vi "test.vi"() -> ()   [LabVIEW 2017]
uses:
  <vilib>/Instr/_visa.llb/VISA Configure Serial Port (Instr).vi
panel:
  out "返回数 2":u32
  out "返回数":u32
  in  "输入串口（com12）":refnum<visa-resource-name>="COM12"
  out "读取缓冲区1":string="i"
  in  "停止":bool
  in  "输出串口（com13）":refnum<visa-resource-name>="COM13"
  in  "输入串口（com11）":refnum<visa-resource-name>="COM11"
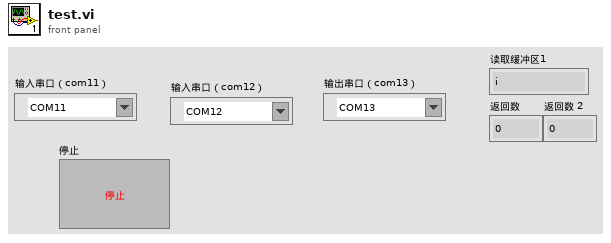
[diagram p1: front panel]
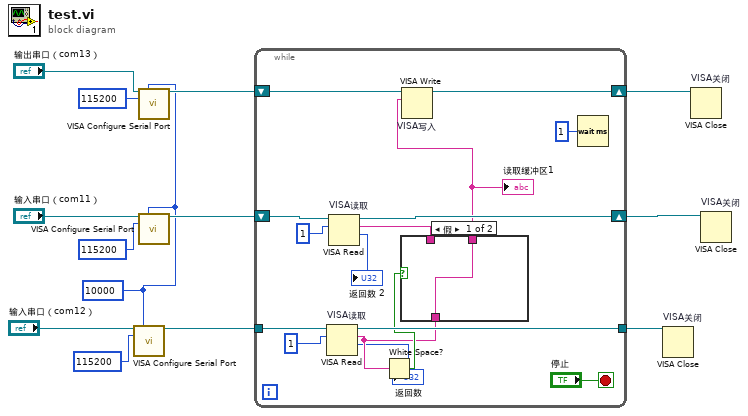
[diagram p0: block diagram]
diagram:
  w1 = u32 10000 ("timeout (10sec)")
  n1 = call-poly "VISA Configure Serial Port"("VISA resource name"="输入串口（com12）", "timeout (10sec)"=w1, "baud rate (9600)"=u32 115200) -> ("VISA resource name out"=w3:refnum<visa-resource-name>)  [unwired: 11 in, 1 out]
  n2 = call-poly "VISA Configure Serial Port"("VISA resource name"="输出串口（com13）", "timeout (10sec)"=w1, "baud rate (9600)"=u32 115200) -> ("VISA resource name out"=w8:refnum<visa-resource-name>)  [unwired: 11 in, 1 out]
  n3 = call-poly "VISA Configure Serial Port"("VISA resource name"="输入串口（com11）", "timeout (10sec)"=w1, "baud rate (9600)"=u32 115200) -> ("VISA resource name out"=w11:refnum<visa-resource-name>)  [unwired: 11 in, 1 out]
  n4 = while {
    shift-right: [w27] -> w7
    shift-left: w11 -> [w29]
    shift-right: [w26] -> w6
    shift-left: w8 -> [w28]
    tunnel: w3 -> [w22]
    tunnel: [w20] -> w2
    stop <- "停止" stop-if-true
    n5 = VISA Read "VISA读取"(VISA resource name=w22, byte count=u32 1 ("字节总数")) -> (VISA resource name out=w20:refnum<visa-resource-name>, read buffer=w17:string, return count=→"返回数":u32)  [unwired: 1 in, 1 out]
    n6 = VISA Read "VISA读取"(VISA resource name=w29, byte count=u32 1 ("字节总数")) -> (VISA resource name out=w27:refnum<visa-resource-name>, read buffer=w21:string, return count=→"返回数 2":u32)  [unwired: 1 in, 1 out]
    n7 = White Space?(1:w17) -> (0:w18:bool)
    n8 = case shown="假" w18 {
      tunnel: w21 -> [_ w31]
      tunnel: [w30 w31] -> w16
      tunnel: w17 -> [w30 _]
      frame False {
      }
      frame True {
      }
    }
    "读取缓冲区1" <- w16
    n9 = VISA Write "VISA写入"(VISA resource name=w28, write buffer=w16) -> (VISA resource name out=w26:refnum<visa-resource-name>)  [unwired: 1 in, 2 out]
    n10 = Wait (ms)(milliseconds to wait=u32 1 ("等待时间（毫秒）")) -> ()  [unwired: 1 out]
  }
  n11 = VISA Close "VISA关闭"(VISA resource name=w2) -> ()  [unwired: 1 in, 1 out]
  n12 = VISA Close "VISA关闭"(VISA resource name=w6) -> ()  [unwired: 1 in, 1 out]
  n13 = VISA Close "VISA关闭"(VISA resource name=w7) -> ()  [unwired: 1 in, 1 out]
